vi "Config File First Hour.vi"(0 "Config File Path":path=path "C:/NI-2010/Trunk/Hybrid Water Heater/HEWH First Hour Rating.ini", 7 "Read/Write Config":bool=TRUE, 11 "Error In":errorcluster) -> (3 "Test Condition Settings Cluster":T3={"Serial Port Available?"=TRUE, "Cold Water Available?"=TRUE, "TempErLimit"=20.0, "Temp Decline Hystersis"=0.2, "Target IP Address"="192.168.25.3", "Draw Tesw Condition"=enum."SRK500,Station1,5GPM FR"}, 4 "DOE Test Spec Settings Cluster":T4={"Degree Setting"=58.0, "Flow rate setting"=3.0, "TFall"=25.0, "End Time(s)"=3600.0, "Tc1 LL"=130.0, "Tc1 UL"=140.0}, 6 "Timing Cluster":T5={"No Serial  Sample Period(s)"=10.0, "T5"=1000, "T4"=60000, "T1"=1000, "T2"=150, "T3"=500}, 8 "Purge Settings Cluster":T6={"Temp SettleTimeLimit(S)"=60.0, "Steady State Persist Time(mS)"=5000, "Purge Min Time"=10000, "Flow SettleTimeLimit(S)"=300.0, "Flow Adjust Time (3s)"=3.0, "Flow Band (+/-GPM)"=0.25, "Proportional Control Adjust Rate"=0.1}, 10 "Purge Condition Settings Cluster":T7={"PurgreTempLimit"=127.0, "Purge Condition TC"=enum."TC1", "Purgre0TempLim"=127.0, "Purge Guard Time(s)"=120.0}, 15 "Error Out":errorcluster)   [LabVIEW 2013]
uses:
  Type Definitions/TestedFlowratesScenarios.ctl
  Type Definitions/Cluster Purge Settings.ctl
  <vilib>/Utility/config.llb/Write Key (Boolean).vi
  <vilib>/Utility/config.llb/Write Key (String).vi
  <vilib>/Utility/config.llb/Write Key (Path).vi
  <vilib>/Utility/config.llb/Write Key (I32).vi
  <vilib>/Utility/config.llb/Write Key (Double).vi
  <vilib>/Utility/config.llb/Read Key (Boolean).vi
  <vilib>/Utility/config.llb/Read Key (String).vi
  <vilib>/Utility/config.llb/Read Key (Path).vi
  <vilib>/Utility/config.llb/Read Key (Double).vi
  <vilib>/Utility/config.llb/Read Key (I32).vi
  <vilib>/Utility/config.llb/NI_LVConfig.lvlib
panel:
  out "Array":string[][](array[string])
  in  "Prompt":string="Enter Filename:"
  in  "Tab Control":T1(tab)
  # "Sample Period for Decision Data"
  # "Loop Delays, prevent overwork Machine"
  # "UI Refresh Rate"
  # "1 Min Between Samps in spec."
  # "Flow Loop Time"
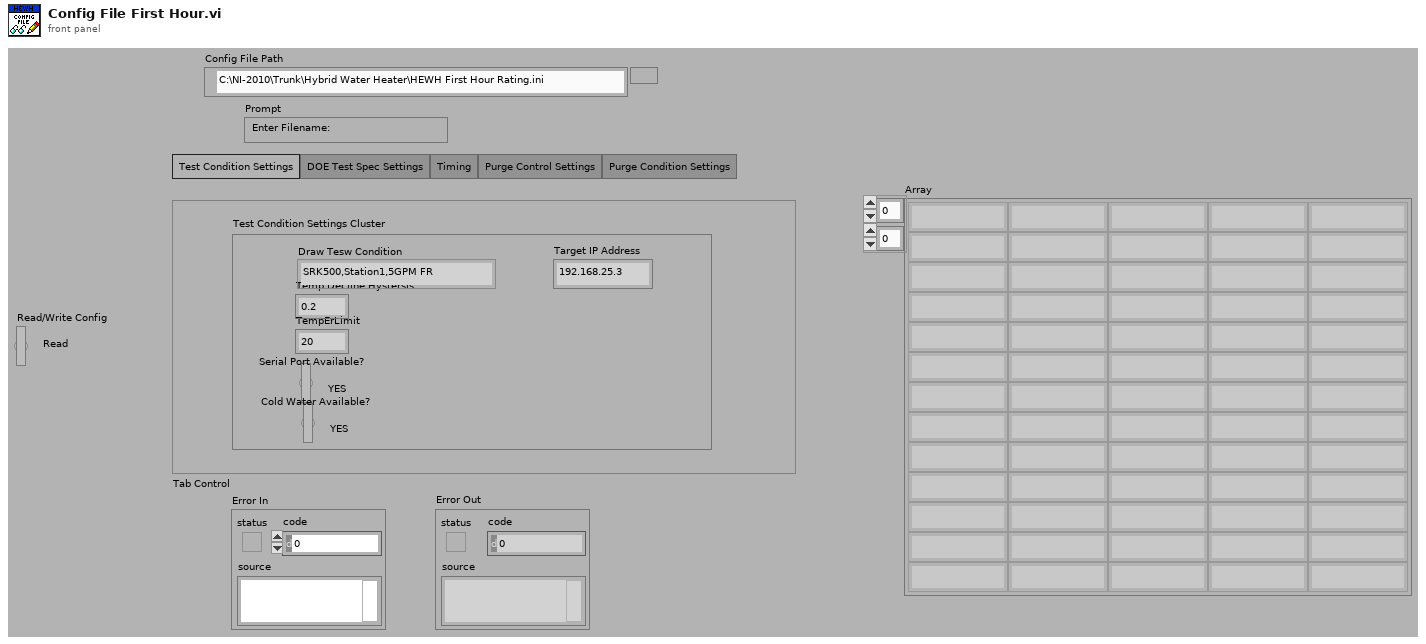
[diagram p1: front panel]
types:
  T1 = enum32{"Test Condition Settings", "DOE Test Spec Settings", "Timing", "Purge Control Settings", "Purge Condition Settings"}
  T2 = typedef "TestedFlowratesScenarios.ctl" = enum16{"DRK500,Station1", "DRK375,Lab", "SRK500,Station1,5GPM FR", "DRK375,STATION3,1/2\"HOSE", "DRK500,Station1,downspout", "DRK375,Station3,thruEcocute", "DRK375,Station3,purge", "Build2,2B,Purge", "Global, Purge", "Global, Tank"}
  T3 = cluster{"Serial Port Available?":bool, "Cold Water Available?":bool, "TempErLimit":dbl, "Temp Decline Hystersis":dbl, "Target IP Address":string, "Draw Tesw Condition":T2}
  T4 = cluster{"Degree Setting":dbl, "Flow rate setting":dbl, "TFall":dbl, "End Time(s)":dbl, "Tc1 LL":dbl, "Tc1 UL":dbl}
  T5 = cluster{"No Serial  Sample Period(s)":dbl, "T5":u32, "T4":u32, "T1":u32, "T2":u32, "T3":u32}
  T6 = typedef "Cluster Purge Settings.ctl" = cluster{"Temp SettleTimeLimit(S)":dbl, "Steady State Persist Time(mS)":u32, "Purge Min Time":i32, "Flow SettleTimeLimit(S)":dbl, "Flow Adjust Time (3s)":dbl, "Flow Band (+/-GPM)":dbl, "Proportional Control Adjust Rate":dbl}
  T7 = cluster{"PurgreTempLimit":dbl, "Purge Condition TC":enum16{"TC1", "TC2", "TC3", "TC4", "TC5", "TC6"}, "Purgre0TempLim":dbl, "Purge Guard Time(s)":dbl}
  T8 = typedef "NI_LVConfig.lvlib/Config Data RefNum.ctl" = refnum<k1>
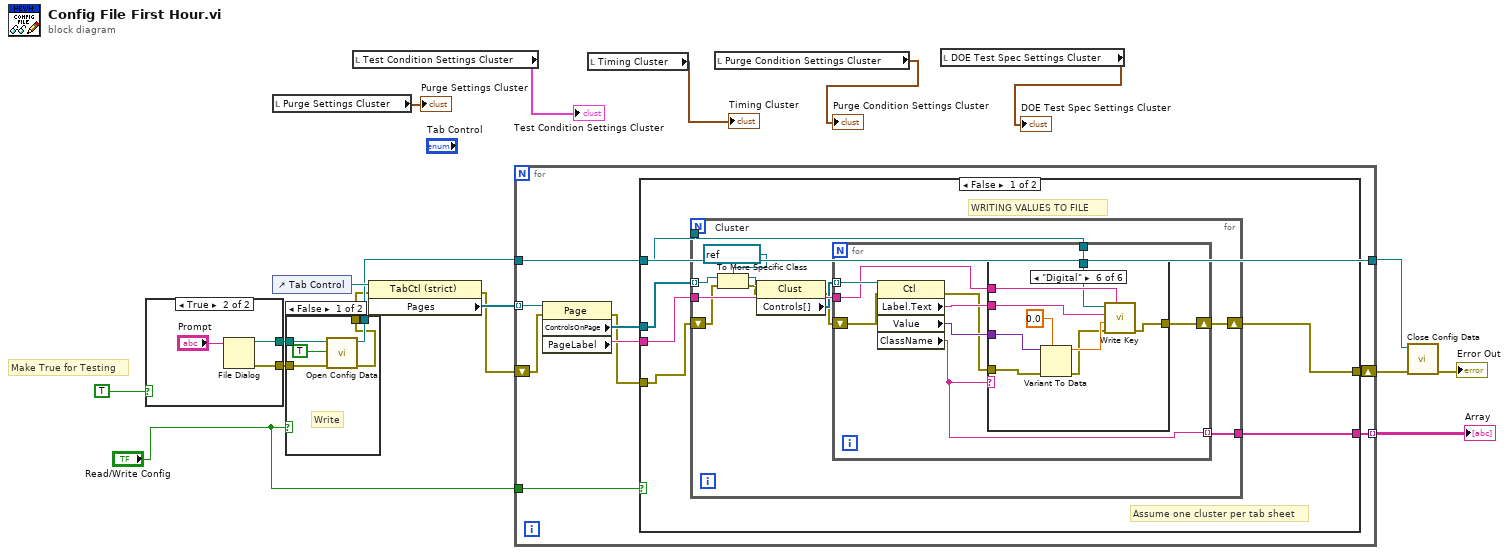
[diagram p0: block diagram]
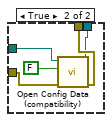
[diagram p2: hidden frame]
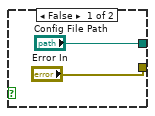
[diagram p3: hidden frame]
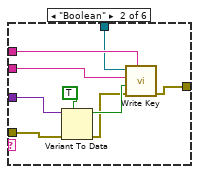
[diagram p5: hidden frame]
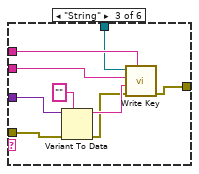
[diagram p6: hidden frame]
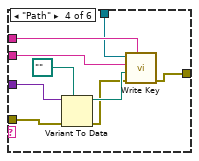
[diagram p7: hidden frame]
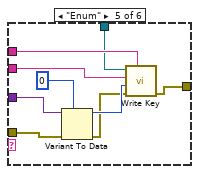
[diagram p8: hidden frame]
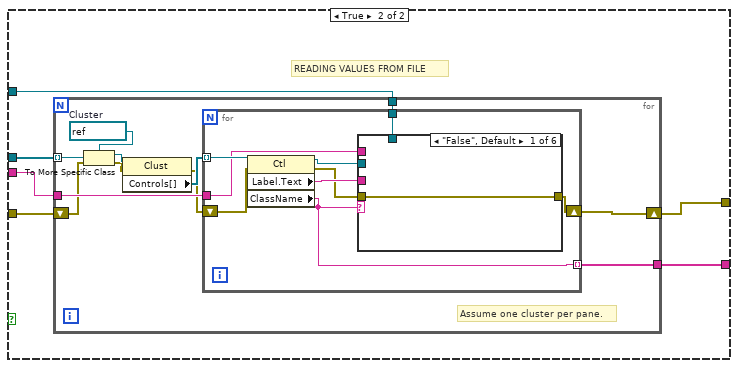
[diagram p9: hidden frame]
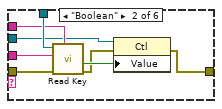
[diagram p10: hidden frame]
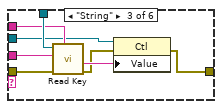
[diagram p11: hidden frame]
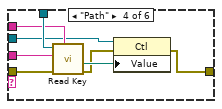
[diagram p12: hidden frame]
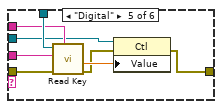
[diagram p13: hidden frame]
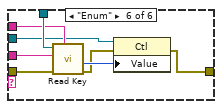
[diagram p14: hidden frame]
diagram:
  # "Make True for Testing"
  n1 = case shown="True" TRUE {
    tunnel: ["Config File Path" w23] -> w16
    tunnel: ["Error In" w21] -> w15
    frame False {
    }
    frame True {
      n2 = File Dialog(7:"Prompt") -> (0:w21:errorcluster, 3:w23:path)  [unwired: 1 in, 7 out]
    }
  }
  n3 = local read "Purge Settings Cluster"() -> (→"Purge Settings Cluster":T6)
  n4 = control-ref of="Tab Control"() -> (w18:refnum<vi>)
  n5 = case shown="False" "Read/Write Config" {
    tunnel: w16 -> [w28 w29]
    tunnel: w15 -> [w27 w32]
    tunnel: [w26 w30] -> w14
    tunnel: [w24 w31] -> w8
    frame False {
      # "Write"
      n6 = call <vilib>:"Open Config Data.vi"("error in (no error)"=w27, "create file if necessary (T)"=TRUE, "configuration file path"=w28) -> ("error out"=w24:errorcluster, "refnum"=w26:T8)  [unwired: 7 out]
    }
    frame True {
      n7 = call <vilib>:"Open Config Data (compatibility).vi"("error in (no error)"=w32, "create file if necessary (T)"=FALSE ("create file if necessary? (T)"), "configuration file path"=w29) -> ("error out"=w31:errorcluster, "refnum"=w30:T8)  [unwired: 6 in, 1 out]
    }
  }
  n8 = local read "Test Condition Settings Cluster"() -> (→"Test Condition Settings Cluster":T3)
  n9 = property class="TabCtl (strict)"(reference=w18, error in=w8) -> (error out=w6:errorcluster, "Pages"=w17:refnum<vi>[])  [unwired: 1 out]
  n10 = for {
    tunnel: w17 -> [w42] mode=indexing
    tunnel: w14 -> [w38]
    tunnel: [w39] -> w13 mode=indexing
    tunnel: [w38] -> w11
    tunnel: "Read/Write Config" -> [w36]
    shift-right: [w37] -> w10
    shift-left: w6 -> [w35]
    n11 = property class="Page"(reference=w42, error in=w35) -> (error out=w34:errorcluster, "ControlsOnPage"=w41:refnum<vi>[], "PageLabel"=w40:string)  [unwired: 1 out]
    n12 = case shown="False" w36 {
      tunnel: w41 -> [w48 w120]
      tunnel: w40 -> [w47 w119]
      tunnel: [w44 w118] -> w39
      tunnel: w38 -> [w46 w117]
      tunnel: [w45 w116] -> w37
      tunnel: w34 -> [w43 w115]
      frame False {
        # "Assume one cluster per tab sheet"
        # "WRITING VALUES TO FILE"
        n13 = for {
          tunnel: w48 -> [w52] mode=indexing
          tunnel: w47 -> [w59]
          tunnel: w46 -> [w58]
          tunnel: [w56] -> w44
          shift-right: [w57] -> w45
          shift-left: w43 -> [w50]
          w55 = refnum<vi> refnum  # Cluster
          n14 = To More Specific Class(target class=w55, reference=w52, error in=w50) -> (specific class reference=w54:refnum<vi>, error out=w53:errorcluster)
          n15 = property class="Clust"(reference=w54, error in=w53) -> (error out=w49:errorcluster, "Controls[]"=w51:refnum<vi>[])  [unwired: 1 out]
          n16 = for {
            tunnel: w51 -> [w68] mode=indexing
            tunnel: w59 -> [w65]
            tunnel: w58 -> [w64]
            tunnel: [w63] -> w56 mode=indexing
            shift-right: [w62] -> w57
            shift-left: w49 -> [w61]
            n17 = property class="Ctl"(reference=w68, error in=w61) -> (error out=w60:errorcluster, "Label.Text"=w67:string, "Value"=w66:variant, "ClassName"=w63:string)  [unwired: 1 out]
            n18 = case shown="\"Digital\"" w63 {
              tunnel: w67 -> [_ w78 w87 w96 w105 w114]
              tunnel: w66 -> [_ w77 w86 w95 w104 w113]
              tunnel: w65 -> [_ w74 w84 w93 w102 w111]
              tunnel: w64 -> [_ w73 w83 w92 w101 w110]
              tunnel: [w69 w72 w82 w91 w100 w109] -> w62
              tunnel: w60 -> [w69 w71 w80 w89 w98 w107]
              frame "False", Default {
              }
              frame "Boolean" {
                n19 = Variant To Data(error in=w71, type=TRUE, Variant=w77) -> (data=w75:bool, error out=w70:errorcluster)
                n20 = call-poly <vilib>:"Write Key.vi"("section"=w74, "error in (no error)"=w70, "value"=w75, "key"=w78, "refnum"=w73) -> ("error out"=w72:errorcluster)  [unwired: 1 in, 5 out]
              }
              frame "String" {
                n21 = Variant To Data(error in=w80, type="", Variant=w86) -> (data=w85:string, error out=w79:errorcluster)
                n22 = call-poly <vilib>:"Write Key.vi"("section"=w84, "error in (no error)"=w79, "value"=w85, "key"=w87, "refnum"=w83) -> ("error out"=w82:errorcluster)  [unwired: 1 in, 5 out]
              }
              frame "Path" {
                n23 = Variant To Data(error in=w89, type=path "", Variant=w95) -> (data=w94:path, error out=w88:errorcluster)
                n24 = call-poly <vilib>:"Write Key.vi"("section"=w93, "error in (no error)"=w88, "value"=w94, "key"=w96, "refnum"=w92) -> ("error out"=w91:errorcluster)  [unwired: 1 in, 5 out]
              }
              frame "Enum" {
                n25 = Variant To Data(error in=w98, type=0, Variant=w104) -> (data=w103:i32, error out=w97:errorcluster)
                n26 = call-poly <vilib>:"Write Key.vi"("section"=w102, "error in (no error)"=w97, "value"=w103, "key"=w105, "refnum"=w101) -> ("error out"=w100:errorcluster)  [unwired: 1 in, 5 out]
              }
              frame "Digital" {
                n27 = Variant To Data(error in=w107, type=0.0, Variant=w113) -> (data=w112:dbl, error out=w106:errorcluster)
                n28 = call-poly <vilib>:"Write Key.vi"("section"=w111, "error in (no error)"=w106, "value"=w112, "key"=w114, "refnum"=w110) -> ("error out"=w109:errorcluster)  [unwired: 3 in, 3 out]
              }
            }
          }
        }
      }
      frame True {
        # "READING VALUES FROM FILE"
        n29 = for {
          tunnel: w120 -> [w127] mode=indexing
          tunnel: w119 -> [w131]
          tunnel: [w130] -> w118
          tunnel: w117 -> [w129]
          shift-right: [w128] -> w116
          shift-left: w115 -> [w123]
          w126 = refnum<vi> refnum  # Cluster
          # "Assume one cluster per pane."
          n30 = To More Specific Class(target class=w126, reference=w127, error in=w123) -> (specific class reference=w125:refnum<vi>, error out=w122:errorcluster)
          n31 = property class="Clust"(reference=w125, error in=w122) -> (error out=w121:errorcluster, "Controls[]"=w124:refnum<vi>[])  [unwired: 1 out]
          n32 = for {
            tunnel: w124 -> [w140] mode=indexing
            tunnel: w131 -> [w138]
            tunnel: w129 -> [w137]
            tunnel: [w135] -> w130 mode=indexing
            shift-right: [w136] -> w128
            shift-left: w121 -> [w133]
            n33 = property class="Ctl"(reference=w140, error in=w133) -> (reference out=w134:refnum<vi>, error out=w132:errorcluster, "Label.Text"=w139:string, "ClassName"=w135:string)
            n34 = case shown="\"False\", Default" w135 {
              tunnel: w139 -> [_ w149 w157 w165 w173 w181]
              tunnel: w138 -> [_ w147 w155 w163 w171 w179]
              tunnel: w137 -> [_ w148 w156 w164 w172 w180]
              tunnel: [w141 w144 w152 w160 w168 w176] -> w136
              tunnel: w134 -> [_ w146 w154 w162 w170 w178]
              tunnel: w132 -> [w141 w142 w150 w158 w166 w174]
              frame "False", Default {
              }
              frame "Boolean" {
                n35 = call-poly <vilib>:"Read Key.vi"("section"=w147, "error in (no error)"=w142, "key"=w149, "refnum"=w148) -> ("error out"=w143:errorcluster, "value"=w145:bool)  [unwired: 1 in, 5 out]
                n36 = property class="Ctl"(reference=w146, error in=w143, "Value"=w145) -> (error out=w144:errorcluster)  [unwired: 1 out]
              }
              frame "String" {
                n37 = call-poly <vilib>:"Read Key.vi"("section"=w155, "error in (no error)"=w150, "key"=w157, "refnum"=w156) -> ("error out"=w151:errorcluster, "value"=w153:string)  [unwired: 2 in, 4 out]
                n38 = property class="Ctl"(reference=w154, error in=w151, "Value"=w153) -> (error out=w152:errorcluster)  [unwired: 1 out]
              }
              frame "Path" {
                n39 = call-poly <vilib>:"Read Key.vi"("section"=w163, "error in (no error)"=w158, "key"=w165, "refnum"=w164) -> ("error out"=w159:errorcluster, "value"=w161:path)  [unwired: 1 in, 5 out]
                n40 = property class="Ctl"(reference=w162, error in=w159, "Value"=w161) -> (error out=w160:errorcluster)  [unwired: 1 out]
              }
              frame "Digital" {
                n41 = call-poly <vilib>:"Read Key.vi"("section"=w171, "error in (no error)"=w166, "key"=w173, "refnum"=w172) -> ("error out"=w167:errorcluster, "value"=w169:dbl)  [unwired: 1 in, 5 out]
                n42 = property class="Ctl"(reference=w170, error in=w167, "Value"=w169) -> (error out=w168:errorcluster)  [unwired: 1 out]
              }
              frame "Enum" {
                n43 = call-poly <vilib>:"Read Key.vi"("section"=w179, "error in (no error)"=w174, "key"=w181, "refnum"=w180) -> ("error out"=w175:errorcluster, "value"=w177:i32)  [unwired: 1 in, 5 out]
                n44 = property class="Ctl"(reference=w178, error in=w175, "Value"=w177) -> (error out=w176:errorcluster)  [unwired: 1 out]
              }
            }
          }
        }
      }
    }
  }
  "Array" <- w13
  n45 = local read "Timing Cluster"() -> (→"Timing Cluster":T5)
  n46 = local read "Purge Condition Settings Cluster"() -> (→"Purge Condition Settings Cluster":T7)
  n47 = local read "DOE Test Spec Settings Cluster"() -> (→"DOE Test Spec Settings Cluster":T4)
  n48 = call <vilib>:"Close Config Data.vi"("error in (no error)"=w10, "refnum"=w11) -> ("error out"=→"Error Out":errorcluster)  [unwired: 1 in, 8 out]
